vi "Generate Report in HTML.vi"(8 "error in (no error)":errorcluster, 10 "Test Info":T1, 11 "Test Data":string[](array[string])) -> (0 "error out":errorcluster)   [LabVIEW 2021, in "User Interface.lvlib"]
uses:
  User Interface.lvlib
  Create Path Command.ctl
  <vilib>/Utility/NIReport.llb/Append Text Table to Report (wrap).vi
  <vilib>/Utility/NIReport.llb/Append Report Text (str wrap).vi
  <vilib>/Utility/NIReport.llb/NI_report.lvclass
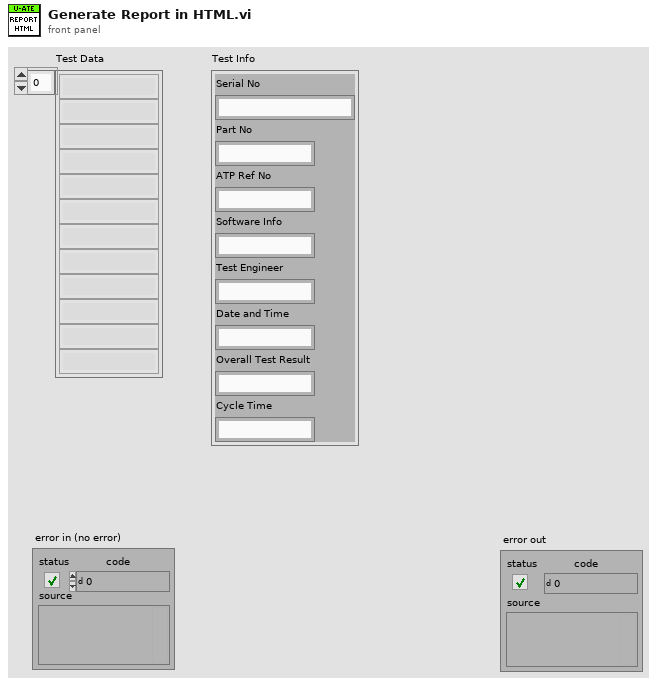
[diagram p1: front panel]
types:
  T1 = cluster{"Serial No":string, "Part No":string, "ATP Ref No":string, "Software Info":string, "Test Engineer":string, "Date and Time":string, "Overall Test Result":string, "Cycle Time":string}
  T2 = enum16{"Standard Report", "HTML", "Word", "Excel"}
  T3 = enum16{"maximized", "minimized", "normal", "no change"}
  T4 = typedef "User Interface.lvlib/Create Path Command.ctl" = enum16{"Authentication", "Hardware", "Configuration", "Calibration", "Instrument", "Test Description", "Serial Data", "Data", "Report", "Action log", "Error Log"}
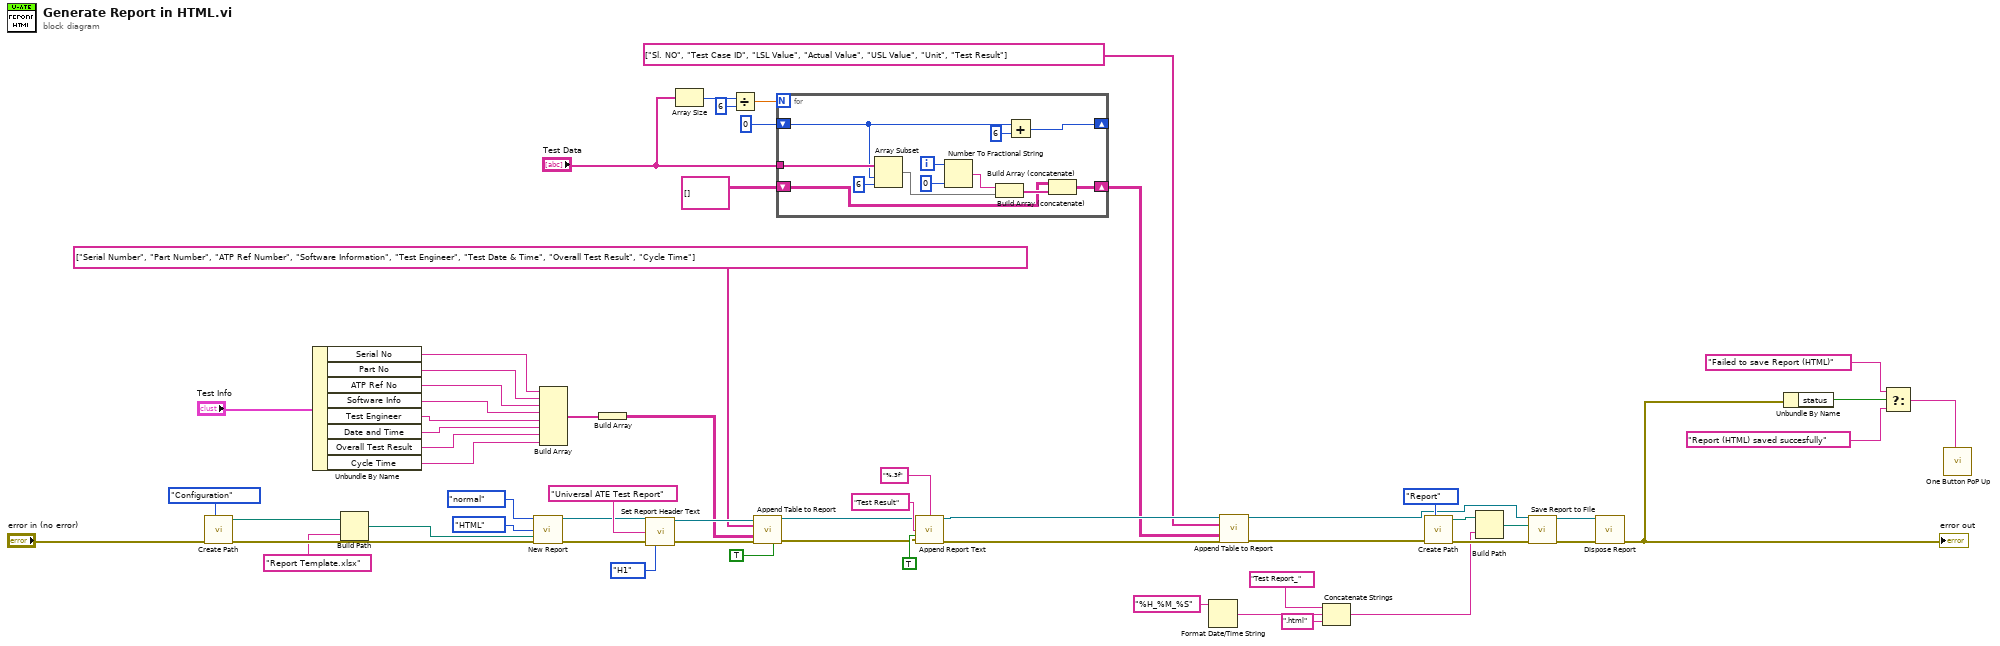
[diagram p0: block diagram]
diagram:
  n1 = call "Create Path.vi"("Path Command"=Create_Path_Command."Configuration", "error in (no error)"="error in (no error)") -> ("error out"=w55:errorcluster, "created path"=w53:path)  [unwired: 8 in]
  n2 = Unbundle By Name("Test Info") -> ("Serial No"=w14:string, "Part No"=w13:string, "ATP Ref No"=w12:string, "Software Info"=w11:string, "Test Engineer"=w10:string, "Date and Time"=w9:string, "Overall Test Result"=w8:string, "Cycle Time"=w7:string)
  n3 = Build Path(base path=w53, name or relative path="Report Template.xlsx") -> (appended path=w60:path)
  n4 = call <vilib>:"New Report.vi"("window state (normal)"=T3."normal", "report type"=T2."HTML", "template (empty)"=w60, "error in (no error)"=w55) -> ("report out"=w25:refnum<class "NI_report.lvclass">, "error out"=w24:errorcluster)  [unwired: 10 in]
  n5 = Build Array(w14, w13, w12, w11, w10, w9, w8, w7) -> (w6:string[])
  n6 = Build Array(w6) -> (w5:string[][])
  n7 = call-dynamic "Set Report Header Text.vi"("report in"=w25, "center header text"="Universal ATE Test Report" ("HEADRER"), "error in (no error)"=w24, "HTML header size"=enum16{"H1", "H2", "H3", "H4", "H5", "H6", "H7"}."H1") -> ("report out"=w22:refnum<class "NI_report.lvclass">, "error out"=w21:errorcluster)  [unwired: 10 in]
  n8 = Array Size(array="Test Data") -> (size(s)=w47:i32)
  n9 = Divide(x=w47, y=6) -> (x/y=w45:dbl)
  n10 = call-poly <vilib>:"Append Table to Report.vi"("report in"=w22, "column headers"=string[] ["Serial Number", "Part Number", "ATP Ref Number", "Software Information", "Test Engineer", "Test Date & Time", "Overall Test Result", "Cycle Time"], "text data"=w5, "error in (no error)"=w21, "show grid lines (YES)"=TRUE) -> ("report out"=w26:refnum<class "NI_report.lvclass">, "error out"=w27:errorcluster)  [unwired: 7 in, 2 out]
  n11 = for {
    N: w45 -> [_]
    shift-right: [w63] -> w18
    shift-left: string[][] [] -> [w61]
    shift-right: [w66] -> _
    shift-left: 0 ("length") -> [w69]
    tunnel: "Test Data" -> [w72]
    i -> [w68]
    n12 = Array Subset(array=w72, index=w69, length=6) -> (w64:string[])
    n13 = Number To Fractional String(number=w68, precision (6)=i16 0) -> (F-format string=w65:string)  [unwired: 2 in]
    n14 = Build Array (concatenate)(w65, w64) -> (w62:string[])
    n15 = Add(x=w69, y=6) -> (x+y=w66:i32)
    n16 = Build Array (concatenate)(w61, w62) -> (w63:string[][])
  }
  n17 = call-poly <vilib>:"Append Report Text.vi"("report in"=w26, "format string (%.3f)"="%.3f", "text"="Test Result", "append on new line? (F)"=TRUE, "error in (no error)"=w27) -> ("report out"=w20:refnum<class "NI_report.lvclass">, "error out"=w19:errorcluster)  [unwired: 7 in, 2 out]
  n18 = Format Date/Time String(time format string (%c)="%H_%M_%S") -> (date/time string=w34:string)  [unwired: 2 in]
  n19 = call-poly <vilib>:"Append Table to Report.vi"("report in"=w20, "column headers"=string[] ["Sl. NO", "Test Case ID", "LSL Value", "Actual Value", "USL Value", "Unit", "Test Result"], "text data"=w18, "error in (no error)"=w19) -> ("report out"=w17:refnum<class "NI_report.lvclass">, "error out"=w16:errorcluster)  [unwired: 8 in, 2 out]
  n20 = Concatenate Strings("Test Report_" ("name or relative path"), w34, ".html" ("string")) -> (w32:string)
  n21 = call "Create Path.vi"("Path Command"=Create_Path_Command."Report", "error in (no error)"=w16) -> ("error out"=w51:errorcluster, "created path"=w50:path)  [unwired: 8 in]
  n22 = Build Path(base path=w50, name or relative path=w32) -> (appended path=w49:path)
  n23 = call-dynamic "Save Report to File.vi"("report in"=w17, "report file path"=w49, "error in (no error)"=w51) -> ("report out"=w58:refnum<class "NI_report.lvclass">, "error out"=w59:errorcluster)  [unwired: 11 in]
  n24 = call-dynamic "Dispose Report.vi"("report in"=w58, "error in (no error)"=w59) -> ("error out"=w39:errorcluster)  [unwired: 13 in]
  "error out" <- w39
  n25 = Unbundle By Name(w39) -> ("status"=w38:bool)
  n26 = Select(t="Failed to save Report (HTML)" ("PopUpText"), s=w38, f="Report (HTML) saved succesfully" ("PopUpText")) -> (s? t:f=w37:string)
  n27 = call "One Button PoP Up.vi"("Message In"=w37) -> ()  [unwired: 11 in]
